vi "CyberSim.vi"() -> ()   [LabVIEW 2014]
doc: "Top-level VI to run one simulation of the iRobot and environment."
uses:
  CyberSim interface/Simulation Configuration.ctl
  autograder/feedbackMode.ctl
  shared/Kobuki Sensor Display.ctl
  shared/Accelerometer.ctl
panel:
  in  "Change Sence":bool
  in  "play":bool
  out "Kobuki Sensors Display":T1={"Center Bump"=FALSE, "Left Wheel Drop"=FALSE, "Right Wheel Drop"=FALSE, "Left Bump"=FALSE, "Right Bump"=FALSE, "Left Cliff"=FALSE, "Center Cliff"=FALSE, "Right Cliff"=FALSE, "Net Dist (mm)"=3605, "Net Angle (deg)"=-38, "Left Cliff"=758, "Center Cliff"=770, "Right Cliff"=758, "Left Wheel (mm/s)"=0, "Right Wheel (mm/s)"=0, "accelerometer"={"x axis (g)"=0.15724706555574047, "y axis (g)"=-0.0026101499423643627, "z axis (g)"=0.9842804420695141}} {"Right Wheel (mm/s)" scale=-500.0..500.0; "Left Wheel (mm/s)" scale=-500.0..500.0}
  in  "check grade":bool
  out "Sequence Number":i32
  in  "home camera":bool
  out "Simulator Display":refnum<vi>(3d-picture)
  out "Simulation Running":bool
  in  "exit":bool=TRUE
  in  "start":bool
  in  "stop":bool
  in  "pause":bool
  in  "Front Panel Tabs":T3(tab)=enum."Configuration"
  out "Statechart Diagram Display (supports LabVIEW Statecharts only)":picture
  out "Feedback":string
  in  "Simulation Configuration":T4={"maxTime"=inf, "enableVisualization"=TRUE, "Environment Definition"=path "Environment - Kobuki Hill Climb 1.xml", "Record Location"=path "Simulation Record.xml", "autograde?"=FALSE, "interactive?"=FALSE, "Feedback Mode"=enum."debug navigation", "Robot State Charts"=[path "../statechart/Simulation Statechart.vi"], "statechart"=path "../statechart/Simulation Statechart.vi"}
  in  "save configuration":bool
  in  "terminate at simulation end?":bool
  in  "Real-Time?":bool
  out "Simulation Time (s)":sgl=48.645 format="%7.3g"
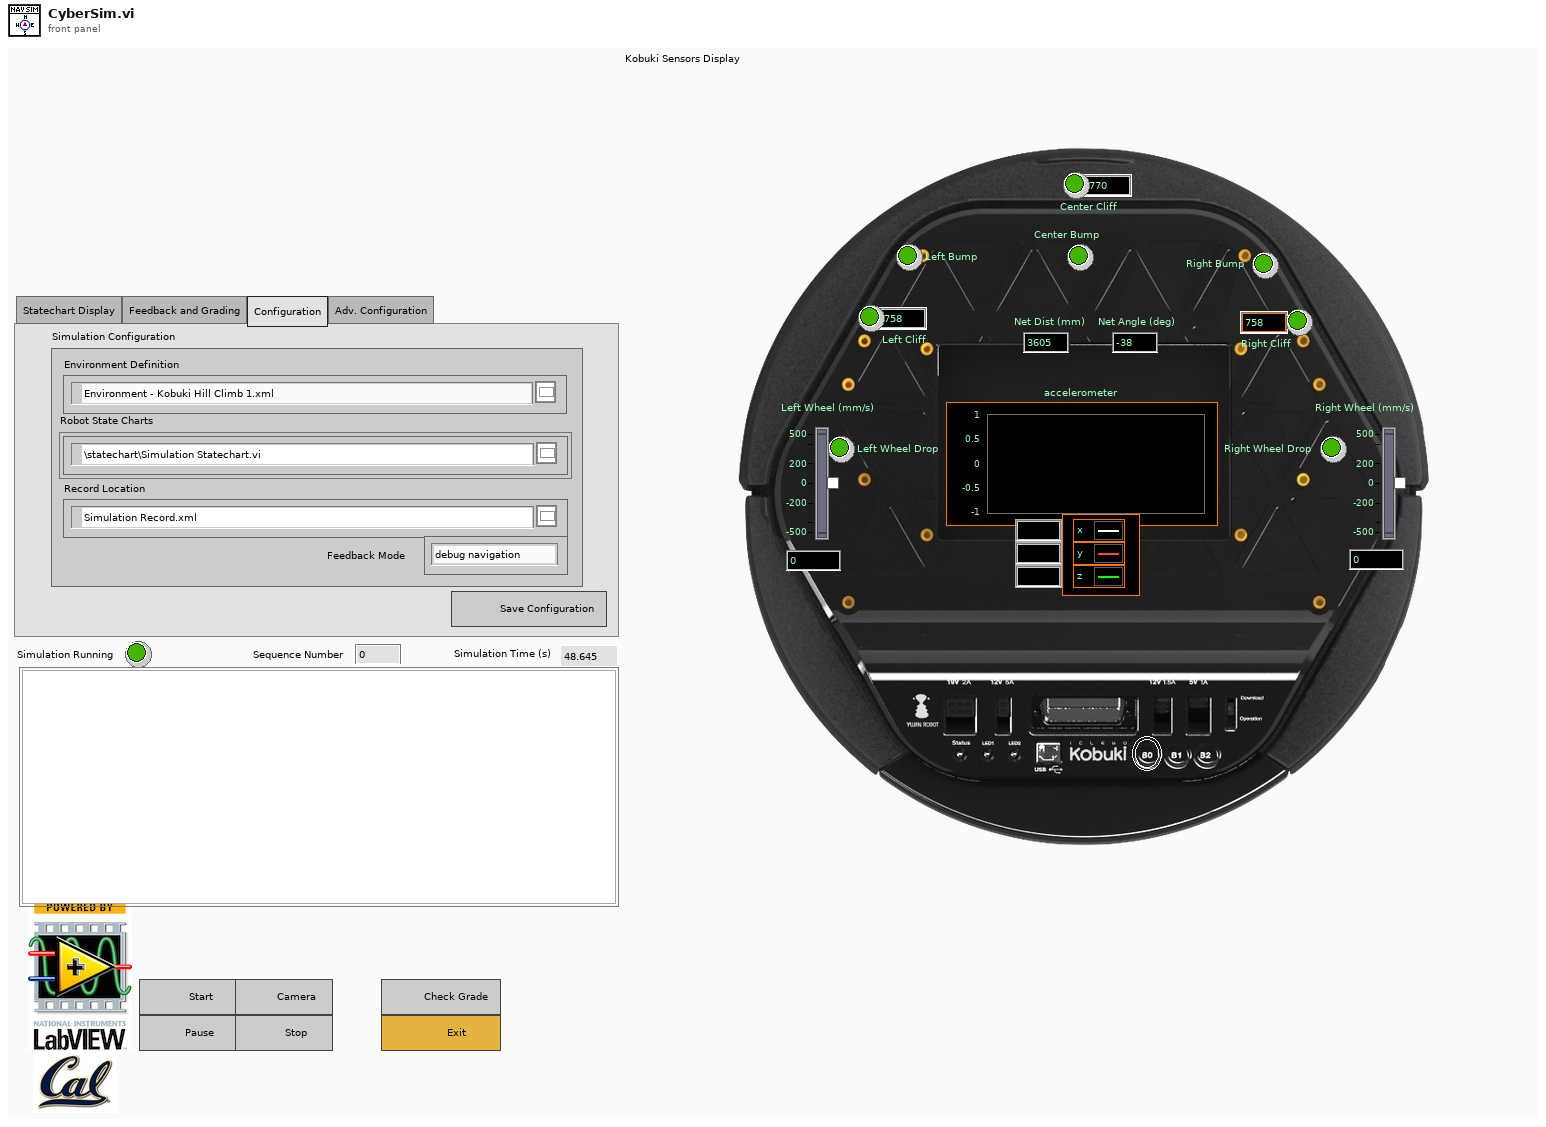
[diagram p1: front panel]
types:
  T1 = typedef "Kobuki Sensor Display.ctl" = cluster{"Center Bump":bool, "Left Wheel Drop":bool, "Right Wheel Drop":bool, "Left Bump":bool, "Right Bump":bool, "Left Cliff":bool, "Center Cliff":bool, "Right Cliff":bool, "Net Dist (mm)":i32, "Net Angle (deg)":i32, "Left Cliff":u16, "Center Cliff":u16, "Right Cliff":u16, "Left Wheel (mm/s)":i16, "Right Wheel (mm/s)":i16, "accelerometer":T2}
  T2 = typedef "Accelerometer.ctl" = cluster{"x axis (g)":dbl, "y axis (g)":dbl, "z axis (g)":dbl}
  T3 = enum32{"Statechart Display", "Feedback and Grading", "Configuration", "Adv. Configuration"}
  T4 = typedef "Simulation Configuration.ctl" = cluster{"maxTime":sgl, "enableVisualization":bool, "Environment Definition":path, "Record Location":path, "autograde?":bool, "interactive?":bool, "Feedback Mode":T5, "Robot State Charts":path[], "statechart":path}
  T5 = typedef "feedbackMode.ctl" = enum32{"debug navigation", "debug hill climb", "autograde navigation", "autograde hill climb"}
  T6 = typedef "Simulator.ctl" = cluster{"configuration":T4, "Statechart\ndisplay":refnum<vi>, "first step?":bool, "Robots Simulation Statecharts":path[], "Robots":T7[]}
  T7 = typedef "RobotData.ctl" = cluster{"Bump Sensors":refnum<k20>[], "Distance Sensors":refnum<k20>[], "Accelerometer":refnum<k20>, "Wall Sensor":refnum<k20>, "Body":refnum<k20>, "RobotID":string, "RobotType":string, "Left Motor":refnum<class "DC Motor Controller.lvclass">, "Right Motor":refnum<class "DC Motor Controller.lvclass">}
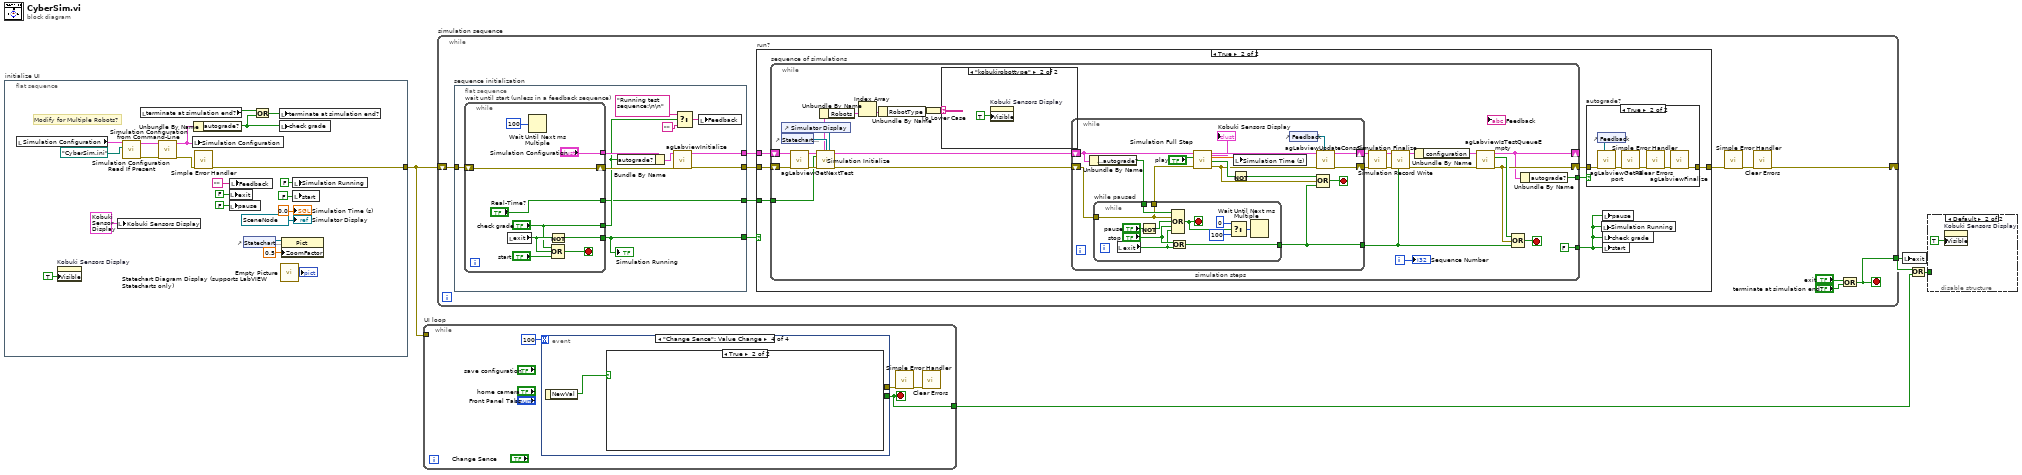
[diagram p0: block diagram]
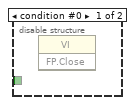
[diagram p2: hidden frame]
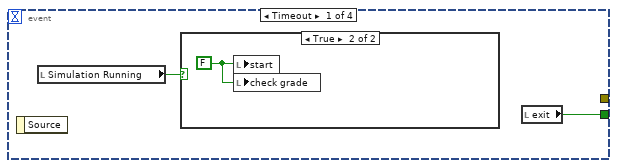
[diagram p3: hidden frame]
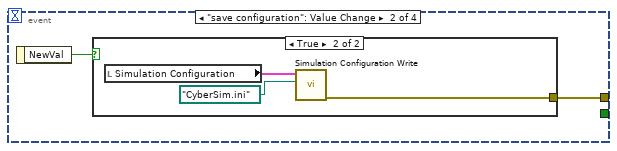
[diagram p5: hidden frame]
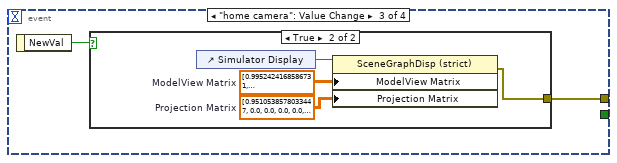
[diagram p7: hidden frame]
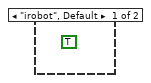
[diagram p12: hidden frame]
diagram:
  n1 = flat-sequence "initialize UI" {
    tunnel: [w23] -> w4
    frame #0 {
      # "Modify for Multiple Robots?"
      n2 = local read "Simulation Configuration"() -> (w21:T4)
      n3 = property on="Kobuki Sensors Display" class="Clust (strict)"("Visible"=TRUE) -> ()  [unwired: 2 in, 2 out]
      n4 = local write "Kobuki Sensors Display"(T1 {"Center Bump"=FALSE, "Left Wheel Drop"=FALSE, "Right Wheel Drop"=FALSE, "Left Bump"=FALSE, "Right Bump"=FALSE, "Left Cliff"=FALSE, "Center Cliff"=FALSE, "Right Cliff"=FALSE, "Net Dist (mm)"=0, "Net Angle (deg)"=0, "Left Cliff"=0, "Center Cliff"=0, "Right Cliff"=0, "Left Wheel (mm/s)"=0, "Right Wheel (mm/s)"=0, "accelerometer"={"x axis (g)"=0.0, "y axis (g)"=0.0, "z axis (g)"=0.0}} ("Kobuki Sensors Display")) -> ()
      n5 = call "Simulation Configuration Read If Present.vi"("configuration"=path "CyberSim.ini", "simulation configuration"=w21) -> ("error out"=w19:errorcluster, "simulation configuration"=w20:T4)  [unwired: 8 in]
      n6 = local read "terminate at simulation end?"() -> (w11:bool)
      n7 = call "Simulation Configuration from Command-Line.vi"("error in"=w19, "simulation configuration in"=w20) -> ("error out"=w18:errorcluster, "simulation configuration out"=w16:T4)  [unwired: 8 in]
      n8 = local write "Simulation Configuration"(w16) -> ()
      n9 = Unbundle By Name(w16) -> ("autograde?"=w10:bool)
      n10 = call <vilib>:"Simple Error Handler.vi"("error in (no error)"=w18) -> ("error out"=w23:errorcluster)  [unwired: 4 in, 4 out]
      n11 = local write "exit"(FALSE ("exit")) -> ()
      n12 = local write "pause"(FALSE ("pause")) -> ()
      n13 = local write "Feedback"("") -> ()
      n14 = control-ref of="Statechart Diagram Display (supports LabVIEW Statecharts only)"() -> (w8:refnum<vi>)
      n15 = Or(x=w11, y=w10) -> (x .or. y?=w12:bool)
      n16 = local write "terminate at simulation end?"(w12) -> ()
      n17 = local write "check grade"(w10) -> ()
      n18 = call "Empty Picture"() -> ("empty picture"=→"Statechart Diagram Display (supports LabVIEW Statecharts only)":picture)
      n19 = property class="Pict"(reference=w8, "ZoomFactor"=sgl 0.5 ("Zoom Factor")) -> ()  [unwired: 1 in, 2 out]
      n20 = local write "Simulation Running"(FALSE ("simulation running")) -> ()
      n21 = local write "start"(FALSE ("start")) -> ()
      "Simulation Time (s)" <- sgl 0.0 ("simulated time (s)")
      "Simulator Display" <- refnum<vi> refnum ("3D Picture")
    }
  }
  n22 = while "UI loop" {
    tunnel: [w28] -> w2
    tunnel: w4 -> [_]
    stop <- w28 stop-if-true
    n23 = event shown="[3] \"Change Sence\": Value Change" {
      selector: _ -> [_ _ _ _]
      dyn-events: _ -> [_ _ _ _]
      timeout: 100 -> [_ _ _ _]
      tunnel: [_ w34 w39 _] -> w29
      tunnel: [w32 _ _ _] -> w28
      event Timeout {
        n24 = event-data() -> ()  [unwired: 1 in, 1 out]
        n25 = local read "Simulation Running"() -> (w31:bool)
        n26 = case shown="True" w31 {
          frame False {
          }
          frame True {
            w33 = FALSE ("AutoGrade")
            n27 = local write "start"(w33) -> ()
            n28 = local write "check grade"(w33) -> ()
          }
        }
        n29 = local read "exit"() -> (w32:bool)
      }
      event "save configuration": Value Change {
        n30 = event-data() -> ("NewVal"=w35:bool)  [unwired: 1 in]
        n31 = case shown="True" w35 {
          tunnel: [_ w37] -> w34
          frame False {
          }
          frame True {
            n32 = local read "Simulation Configuration"() -> (w38:T4)
            n33 = call "Simulation Configuration Write.vi"("configuration"=path "CyberSim.ini", "simulation configuration"=w38) -> ("error out"=w37:errorcluster)  [unwired: 9 in]
          }
        }
      }
      event "home camera": Value Change {
        n34 = event-data() -> ("NewVal"=w40:bool)  [unwired: 1 in]
        n35 = case shown="True" w40 {
          tunnel: [_ w41] -> w39
          frame False {
          }
          frame True {
            w42 = sgl[][] [[0.95105386, 0.0, 0.0, 0.0], [0.0, 2.4142137, 0.0, 0.0], [0.0, 0.0, -1.0002, -0.020002], [0.0, 0.0, -1.0, 0.0]]  # Projection Matrix
            w43 = sgl[][] [[0.9952424, -0.09162651, 0.033122927, -2.4552457], [0.010721975, 0.44090375, 0.8974903, -1.0543748], [-0.09683793, -0.8928653, 0.43978852, -0.9396557], [0.0, 0.0, 0.0, 1.0]]  # ModelView Matrix
            n36 = control-ref of="Simulator Display"() -> (w44:refnum<vi>)
            n37 = property class="SceneGraphDisp (strict)"(reference=w44, "ModelView Matrix"=w43, "Projection Matrix"=w42) -> (error out=w41:errorcluster)  [unwired: 1 in, 1 out]
          }
        }
      }
      event "Change Sence": Value Change {
        n38 = event-data() -> ("NewVal"=w45:bool)  [unwired: 1 in]
        n39 = case shown="True" w45 {
          frame False {
          }
          frame True {
          }
        }
      }
    }
    n40 = call <vilib>:"Simple Error Handler.vi"("error in (no error)"=w29) -> ("error out"=w27:errorcluster)  [unwired: 4 in, 4 out]
    n41 = call <vilib>:"Clear Errors.vi"("error in (no error)"=w27) -> ()  [unwired: 5 in, 2 out]
  }
  n42 = while "simulation sequence" {
    tunnel: [w53] -> w3
    shift-right: [w51] -> _
    shift-left: w4 -> [w47]
    stop <- w53 stop-if-true
    n43 = flat-sequence "sequence initialization" {
      tunnel: [w137] -> w52
      tunnel: [w138] -> w50
      tunnel: [w133] -> w49
      tunnel: w47 -> [w136]
      tunnel: [w128] -> w46
      frame #0 {
        n44 = while "wait until start (unless in a feedback sequence)" {
          shift-right: [w144] -> w135
          shift-left: w136 -> [w144]
          tunnel: ["check grade"] -> w132
          tunnel: ["Simulation Configuration"] -> w134
          tunnel: [w141] -> w133
          tunnel: ["Real-Time?"] -> w128
          stop <- w148 stop-if-true
          n45 = local read "exit"() -> (w147:bool)
          n46 = Wait Until Next ms Multiple(millisecond multiple=u32 100) -> ()  [unwired: 1 out]
          n47 = Not(x=w147) -> (.not. x?=w141:bool)
          n48 = Compound Arithmetic op=OR("check grade", w147, "start") -> (w148:bool)
        }
        "Simulation Running" <- w133
        n49 = Bundle By Name(cluster=w134, "autograde?"=w132) -> (w139:T4)
        n50 = call "agLabviewInitialize.vi"("Error In"=w135, "simulation configuration"=w139) -> ("Error Out"=w138:errorcluster, "simulation configuration"=w137:T4)  [unwired: 8 in]
        n51 = Select(t="Running test sequence:\n\n", s=w132, f="") -> (s? t:f=w130:string)
        n52 = local write "Feedback"(w130) -> ()
      }
    }
    n53 = case "run?" shown="True" w49 {
      tunnel: w52 -> [_ w64]
      tunnel: w50 -> [w57 w63]
      tunnel: [w57 w60] -> w48
      tunnel: w46 -> [_ w58]
      frame False {
      }
      frame True {
        n54 = while "sequence of simulations" {
          shift-right: [w88] -> w61
          shift-left: w63 -> [w83]
          shift-right: [w78] -> _
          shift-left: w64 -> [w82]
          tunnel: [w87] -> w62
          tunnel: [FALSE] -> w59
          tunnel: w58 -> [w77]
          i -> [w99]
          stop <- w98 stop-if-true
          n55 = control-ref of="Simulator Display"() -> (w94:refnum<vi>)
          n56 = control-ref of="Statechart Diagram Display (supports LabVIEW Statecharts only)"() -> (w96:refnum<vi>)
          n57 = call "agLabviewGetNextTest.vi"("Error In"=w83, "simulation configuration"=w82) -> ("Error Out"=w84:errorcluster, "simulation configuration"=w85:T4)  [unwired: 8 in]
          n58 = call "Simulation Initialize.vi"("simulation configuration"=w85, "Statechart display"=w96, "Simulator display"=w94, "Real Time"=w77, "Error In"=w84) -> ("simulator"=w76:T6, "Error Out"=w97:errorcluster)  [unwired: 9 in]
          n59 = Unbundle By Name(w76) -> ("Robots"=w75:T7[])
          n60 = Index Array(array=w75) -> (element=w74:T7)  [unwired: 1 in]
          n61 = Unbundle By Name(w74) -> ("RobotType"=w73:string)
          n62 = To Lower Case(string=w73) -> (all lower case string=w72:string)
          n63 = case shown="\"kobukirobottype\"" w72 {
            frame "irobot", Default {
              (unwired) TRUE ("Visible")
            }
            frame "kobukirobottype" {
              n64 = property on="Kobuki Sensors Display" class="Clust (strict)"("Visible"=TRUE) -> ()  [unwired: 2 in, 2 out]
            }
          }
          n65 = while "simulation steps" {
            shift-right: [w104] -> w93
            shift-left: w76 -> [w110]
            shift-right: [w103] -> w95
            shift-left: w97 -> [w108]
            tunnel: [w111] -> w89
            stop <- w115 stop-if-true
            n66 = Unbundle By Name(w110) -> ("configuration.autograde?"=w109:bool)
            n67 = while "while paused" {
              tunnel: [w123] -> w111
              tunnel: w108 -> [w117]
              tunnel: w109 -> [w118]
              tunnel: [w117] -> w107
              stop <- w119 stop-if-true
              n68 = local read "exit"() -> (w124:bool)
              n69 = Not(x="pause") -> (.not. x?=w126:bool)
              n70 = Or(x="stop", y=w124) -> (x .or. y?=w123:bool)
              n71 = Compound Arithmetic op=OR(w118, w117, w126, "stop", w124) -> (w119:bool)
              n72 = Select(t=u32 0 ("millisecond multiple"), s=w119, f=u32 100 ("millisecond multiple")) -> (s? t:f=w122:u32)
              n73 = Wait Until Next ms Multiple(millisecond multiple=w122) -> ()  [unwired: 1 out]
            }
            n74 = call "Simulation Full Step.vi"("Error In"=w107, "Play Button (false)"="play", "simulator"=w110) -> ("Error Out"=w106:errorcluster, "continue to next step?"=w116:bool, "simulated time (s)"=w113:sgl, "simulator"=w105:T6, "Kobuki Sensors Display"=→"Kobuki Sensors Display":T1)  [unwired: 4 in]
            n75 = Not(x=w116) -> (.not. x?=w112:bool)
            n76 = local write "Simulation Time (s)"(w113) -> ()
            n77 = control-ref of="Feedback"() -> (w102:refnum<vi>)
            n78 = call "agLabviewUpdateConsole.vi"("console"=w102, "Error In"=w106, "simulator"=w105) -> ("Error Out"=w103:errorcluster, "simulator"=w104:T6)  [unwired: 7 in]
            n79 = Compound Arithmetic op=OR(w112, w106, w111) -> (w115:bool)
          }
          n80 = call "Simulation Record Write.vi"("Error In"=w95, "simulator"=w93) -> ("Error Out"=w91:errorcluster, "simulator"=w92:T6)  [unwired: 8 in]
          n81 = call "Simulation Finalize.vi"("terminated by user?"=w89, "error in (no error)"=w91, "simulator"=w92) -> ("error out"=w80:errorcluster, "simulator"=w81:T6)  [unwired: 7 in]
          n82 = Unbundle By Name(w81) -> ("configuration"=w79:T4)
          n83 = call "agLabviewIsTestQueueEmpty.vi"("Error In"=w80, "simulation configuration"=w79) -> ("Error Out"=w88:errorcluster, "Empty?"=w90:bool, "simulation configuration"=w78:T4)  [unwired: 7 in]
          n84 = Compound Arithmetic op=OR(w90, w88, w89) -> (w98:bool)
          n85 = Unbundle By Name(w78) -> ("autograde?"=w87:bool)
          "Sequence Number" <- w99
        }
        n86 = case "autograde?" shown="True" w62 {
          tunnel: [w65 w71] -> w60
          tunnel: w61 -> [w65 w70]
          frame False {
          }
          frame True {
            n87 = control-ref of="Feedback"() -> (w69:refnum<vi>)
            n88 = call "agLabviewGetReport.vi"("console"=w69, "Error In"=w70) -> ("Error Out"=w67:errorcluster)  [unwired: 9 in]
            n89 = call <vilib>:"Simple Error Handler.vi"("error in (no error)"=w67) -> ("error out"=w68:errorcluster)  [unwired: 4 in, 4 out]
            n90 = call <vilib>:"Clear Errors.vi"("error in (no error)"=w68) -> ("error out"=w66:errorcluster)  [unwired: 5 in, 1 out]
            n91 = call "agLabviewFinalize.vi"("Error In"=w66) -> ("Error Out"=w71:errorcluster)  [unwired: 10 in]
          }
        }
        n92 = local write "Simulation Running"(w59) -> ()
        n93 = local write "pause"(w59) -> ()
        n94 = local write "check grade"(w59) -> ()
        n95 = local write "start"(w59) -> ()
      }
    }
    n96 = call <vilib>:"Simple Error Handler.vi"("error in (no error)"=w48) -> ("error out"=w56:errorcluster)  [unwired: 4 in, 4 out]
    n97 = call <vilib>:"Clear Errors.vi"("error in (no error)"=w56) -> ("error out"=w51:errorcluster)  [unwired: 5 in, 1 out]
    n98 = Or(x="exit", y="terminate at simulation end?") -> (x .or. y?=w53:bool)
  }
  n99 = local write "exit"(w3) -> ()
  n100 = Or(x=w3, y=w2) -> (x .or. y?=w1:bool)
  n101 = disable-structure shown="Default" {
    disable-tunnel: w1 -> [_ _]
    frame condition #0 {
      n102 = invoke class="VI" method="FP.Close"() -> ()  [unwired: 3 in, 3 out]
    }
    frame condition #1 (active) {
      n103 = property on="Kobuki Sensors Display" class="Clust (strict)"("Visible"=TRUE) -> ()  [unwired: 2 in, 2 out]
    }
  }
